vi "niDTS GNSS GPS Rx RF Test Close.vi"(0 "Template Tx Test Handle":T1, 11 "error in (no error)":errorcluster) -> (15 "error out":errorcluster)   [LabVIEW 2014, in "niDTS GNSS.lvlib"]
uses:
  niDTS GNSS.lvlib
  RF Test/Includes/niDTS GNSS RF Test INC Handle.ctl
  RF Test/Objects/BASE_class/niDTS GNSS RF Test.lvclass
  Framework/Session/Includes/niDTS Session INC Force Destroy.ctl
  Framework/niDTS Framework.lvlib
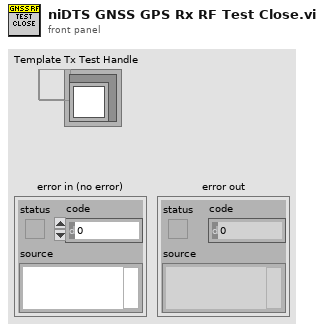
[diagram p1: front panel]
types:
  T1 = typedef "niDTS GNSS.lvlib/niDTS GNSS RF Test INC Handle.ctl" = refnum<data-value>
  T2 = typedef "niDTS Framework.lvlib/niDTS Session INC Force Destroy.ctl" = bool
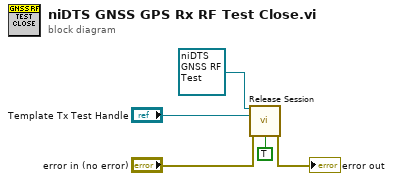
[diagram p0: block diagram]
diagram:
  n1 = call-dynamic "Release Session.vi"("OBJ - Session in"=refnum<class "niDTS GNSS RF Test.lvclass"> refnum ("Template.lvlib:Template Tx Test.lvclass"), "Session Handle in"="Template Tx Test Handle", "error in (no error)"="error in (no error)", "Force Destroy? (F)"=T2 TRUE) -> ("error out"=→"error out":errorcluster)  [unwired: 10 in, 1 out]
